vi "diagStackMat.vi"(9 "A1":dbl[][](array[numeric]), 11 "A0":dbl[][](array[numeric])) -> (3 "Diag Stack Matrix":dbl[][](array[numeric]))   [LabVIEW 2016]
doc: "Stack the matrixes (2D arrays actually) in the diagonal direction. For the inputs A1 and A2, the output matrix is:\n[A0, 0;\n 0, A1]."
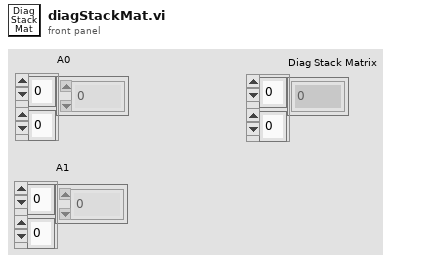
[diagram p1: front panel]
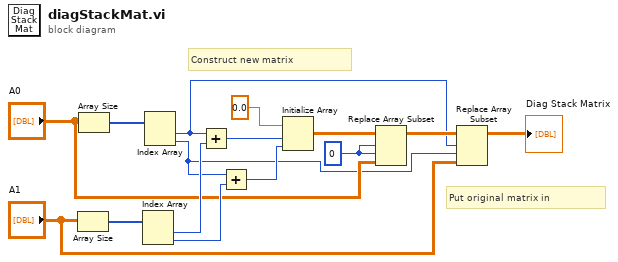
[diagram p0: block diagram]
diagram:
  w7 = 0 ("index (row)")
  # "Put original matrix in"
  # "Construct new matrix"
  n1 = Array Size(array="A1") -> (size(s)=w14:i32[])
  n2 = Array Size(array="A0") -> (size(s)=w15:i32[])
  n3 = Index Array(array=w14) -> (element #1=w13:i32, element #2=w12:i32)  [unwired: 2 in]
  n4 = Index Array(array=w15) -> (element #1=w4:i32, element #2=w3:i32)  [unwired: 2 in]
  n5 = Add(x=w4, y=w13) -> (x+y=w10:i32)
  n6 = Add(x=w3, y=w12) -> (x+y=w9:i32)
  n7 = Initialize Array(0.0 ("element"), w10, w9) -> (w8:dbl[][])
  n8 = Replace Array Subset(array=w8, new element="A0", index (row)=w7, index (col)=w7) -> (w5:dbl[][])
  n9 = Replace Array Subset(array=w5, new element="A1", index (row)=w4, index (col)=w3) -> (→"Diag Stack Matrix":dbl[][])
